vi "Enqueue Message.vi"(8 "error in":errorcluster, 10 "command":T1, 11 "lia host in":refnum<class "LIA Host Interface RT.lvclass">) -> (0 "error out":errorcluster, 3 "lia host out":refnum<class "LIA Host Interface RT.lvclass">)   [LabVIEW 2017, in "LIA Host Interface RT.lvclass"]
uses:
  LIA Host Interface RT.lvclass
  shared/Public/message.ctl
  Properties/OutgoingQueue_GET.vi
  shared/Lock-In Amplifier Example Shared.lvlib
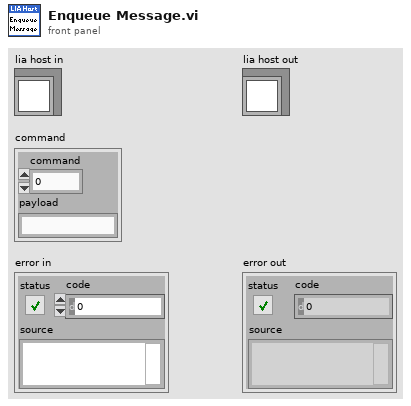
[diagram p1: front panel]
types:
  T1 = typedef "Lock-In Amplifier Example Shared.lvlib/message.ctl" = cluster{"command":u32, "payload":string}
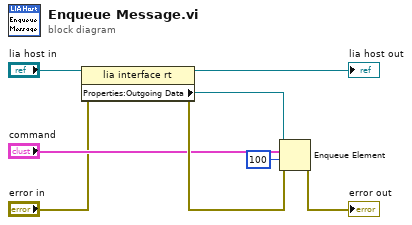
[diagram p0: block diagram]
diagram:
  n1 = property class="lia interface rt"(reference="lia host in", error in="error in") -> (reference out=→"lia host out":refnum<class "LIA Host Interface RT.lvclass">, error out=w6:errorcluster, "Properties:Outgoing Data"=w4:refnum<queue>)
  n2 = Enqueue Element(queue=w4, element="command", timeout in ms (-1)=100, error in (no error)=w6) -> (error out=→"error out":errorcluster)  [unwired: 2 out]
